vi "Channel RepCap.vi"(0 "Channel In":i32) -> (1 "In Range?":bool, 2 "Channel Out":string)   [LabVIEW 2015, in "Rohde&Schwarz CMXP Base.lvlib"]
uses:
  <instrlib>/Rohde&Schwarz CMXP Base/Rohde&Schwarz CMXP Base.lvlib
  <instrlib>/Rohde&Schwarz CMXP Base/Public/Utility/rsidr_core_global.vi
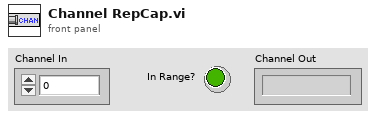
[diagram p1: front panel]
types:
  T1 = typedef "Rohde&Schwarz CMXP Base.lvlib/rsidr_core.lvlib/type_Input_Format_RepCap.ctl" = cluster{"repCapName":string, "indetifiers":string[], "cmdValues":string[]}
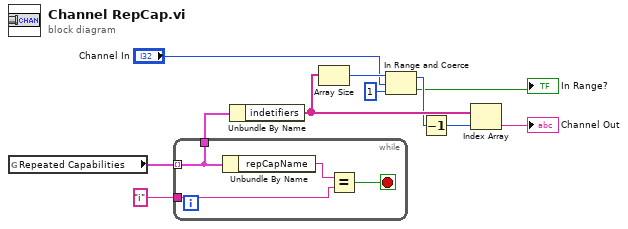
[diagram p0: block diagram]
diagram:
  n1 = global read "rsidr_core_global.vi" "Repeated Capabilities"() -> (w11:T1[])
  n2 = while {
    tunnel: w11 -> [w12] mode=indexing
    tunnel: "i" -> [w14]
    tunnel: [w12] -> w9
    stop <- w13 stop-if-true
    n3 = Unbundle By Name(w12) -> ("repCapName"=w15:string)
    n4 = Equal?(x=w15, y=w14) -> (x = y?=w13:bool)
  }
  n5 = Unbundle By Name(w9) -> ("indetifiers"=w5:string[])
  n6 = Array Size(array=w5) -> (size(s)=w7:i32)
  n7 = In Range and Coerce(upper limit=w7, x="Channel In", lower limit=1) -> (coerced(x)=w4:i32, In Range?=→"In Range?":bool)
  n8 = Decrement(x=w4) -> (x-1=w3:i32)
  n9 = Index Array(array=w5, index=w3) -> (element=→"Channel Out":string)
